vi "pushbutton_switching.vi"() -> ()   [LabVIEW 2011]
panel:
  out "Boolean":bool
  in  "OK Button":bool
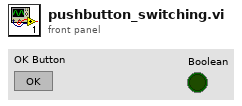
[diagram p1: front panel]
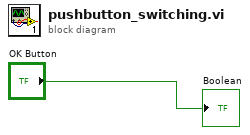
[diagram p0: block diagram]
diagram:
  "Boolean" <- "OK Button"
